vi "test Times Out If One Future Doesnt Resolve.vi"(8 "error in (no error)":errorcluster, 11 "TestCase in":refnum<class "Wait On All Future Tests.lvclass">) -> (0 "error out":errorcluster, 3 "TestCase out":refnum<class "Wait On All Future Tests.lvclass">)   [LabVIEW 2017, in "Wait On All Future Tests.lvclass"]
uses:
  Wait On All Future Tests.lvclass
  <vilib>/addons/_JKI Toolkits/VI Tester/TestCase.llb/TestCase.lvclass
  Futures/Futures.lvlib
  Futures/Promise/Promise.lvclass
  Futures/Future/Future.lvclass
  C:/Program Files (x86)/National Instruments/LabVIEW 2017/vi.lib/addons/_JKI Toolkits/VI Tester/TestCase.llb/TestCase.lvclass
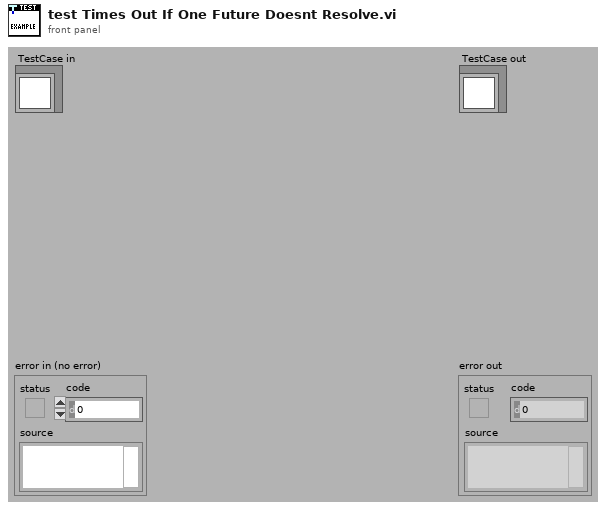
[diagram p1: front panel]
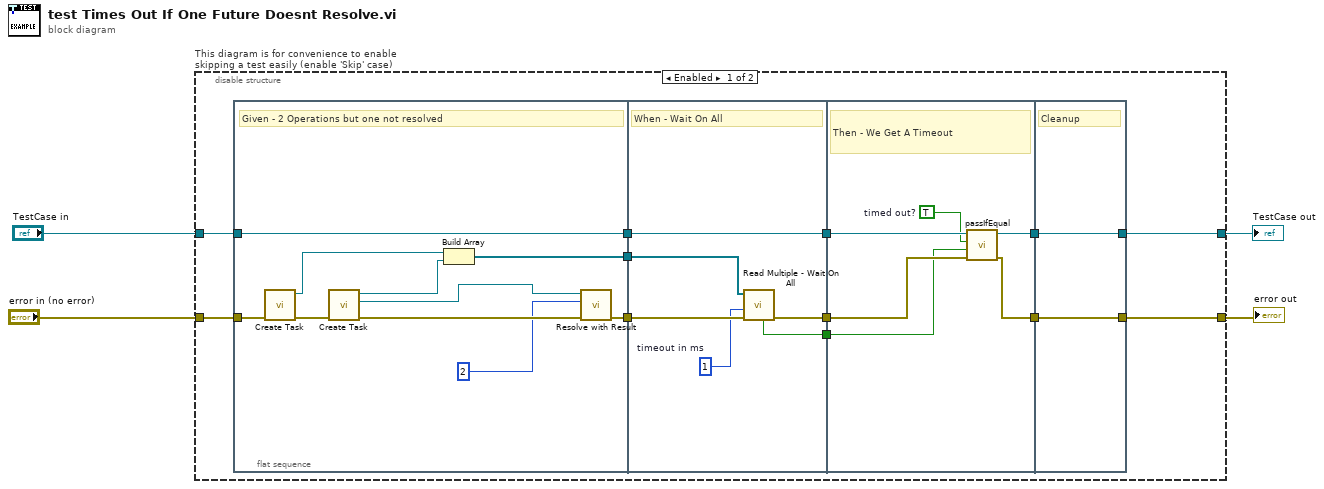
[diagram p0: block diagram]
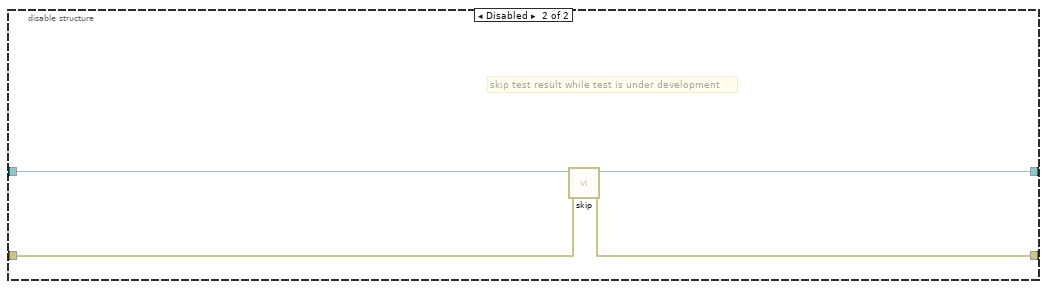
[diagram p2: hidden frame]
diagram:
  n1 = disable-structure "This diagram is for convenience to enable skipping a test easily (enable 'Skip' case)" shown="Enabled" {
    disable-tunnel: "TestCase in" -> [w12 w44]
    disable-tunnel: [w10 w42] -> w1
    disable-tunnel: [w9 w43] -> w3
    disable-tunnel: "error in (no error)" -> [w11 w41]
    frame Enabled {
      n2 = flat-sequence {
        tunnel: w11 -> [w25]
        tunnel: w12 -> [w26]
        tunnel: [w26] -> w16
        tunnel: [w19] -> w7
        tunnel: [w18] -> w6
        tunnel: [w32] -> w15
        tunnel: w16 -> [w32]
        tunnel: [w31] -> w8
        tunnel: w7 -> [w30]
        tunnel: w6 -> [w29]
        tunnel: [w27] -> w5
        tunnel: [w37] -> w14
        tunnel: [w36] -> w13
        tunnel: w15 -> [w38]
        tunnel: w8 -> [w35]
        tunnel: w5 -> [w34]
        tunnel: [w39] -> w9
        tunnel: [w40] -> w10
        tunnel: w14 -> [w40]
        tunnel: w13 -> [w39]
        frame #0 {
          # "Given - 2 Operations but one not resolved"
          n3 = call "Create Task.vi"("error in (no error)"=w25) -> ("error out"=w24:errorcluster, "Future out"=w22:refnum<class "Future.lvclass">)  [unwired: 8 in, 1 out]
          n4 = call "Create Task.vi"("error in (no error)"=w24) -> ("error out"=w21:errorcluster, "Promise out"=w20:refnum<class "Promise.lvclass">, "Future out"=w23:refnum<class "Future.lvclass">)  [unwired: 8 in]
          n5 = Build Array(w22, w23) -> (w19:refnum<class "Future.lvclass">[])
          n6 = call "Resolve with Result.vi"("error in (no error)"=w21, "Result"=2, "Promise in"=w20) -> ("error out"=w18:errorcluster)  [unwired: 8 in]
        }
        frame #1 {
          w28 = 1  # timeout in ms
          # "When - Wait On All"
          n7 = call "Read Multiple - Wait On All.vi"("error in (no error)"=w29, "timeout in ms (60 sec)"=w28, "Futures in"=w30) -> ("error out"=w31:errorcluster, "timed out?"=w27:bool)  [unwired: 5 in, 2 out]
        }
        frame #2 {
          w33 = TRUE  # timed out?
          # "Then - We Get A Timeout"
          n8 = call-dynamic "passIfEqual.vi"("error in (no error)"=w35, "y"=w34, "x"=w33, "TestCase in"=w38) -> ("error out"=w36:errorcluster, "TestCase out"=w37:refnum<class "Wait On All Future Tests.lvclass">)  [unwired: 6 in]
        }
        frame #3 {
          # "Cleanup"
        }
      }
    }
    frame Disabled {
      # "skip test result while test is under development"
      n9 = call <vilib>:"skip.vi"("error in (no error)"=w41, "TestCase in"=w44) -> ("error out"=w43:errorcluster, "TestCase out"=w42:refnum<class "Wait On All Future Tests.lvclass">)  [unwired: 8 in]
    }
  }
  "error out" <- w3
  "TestCase out" <- w1
